vi "sv_Convert Timestamp to Relative Index.vi"(7 "waveform dt":dbl, 10 "timestamp":timestamp, 11 "waveform timestamp":timestamp) -> (2 "Y index":i32)   [LabVIEW 2017]
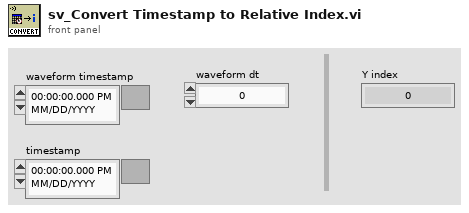
[diagram p1: front panel]
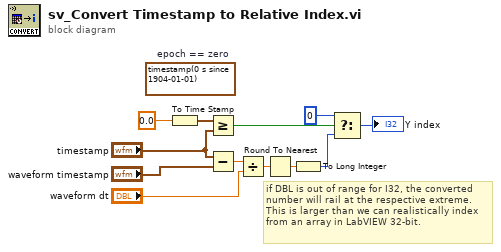
[diagram p0: block diagram]
diagram:
  (unwired) timestamp(0 s since 1904-01-01)  # epoch == zero
  # "if DBL is out of range for I32, the converted number will rail at the respective extreme. This is larger than we can realistically index from an array in LabVIEW 32-bit."
  n1 = To Time Stamp(1:0.0 ("number")) -> (0:w1:timestamp)
  n2 = Greater Or Equal?(x=w1, y="timestamp") -> (x >= y?=w11:bool)
  n3 = Subtract(x="timestamp", y="waveform timestamp") -> (x-y=w7:dbl)
  n4 = Divide(x=w7, y="waveform dt") -> (x/y=w10:dbl)
  n5 = Round To Nearest(number=w10) -> (nearest integer value=w9:dbl)
  n6 = To Long Integer(number=w9) -> (32bit integer=w6:i32)
  n7 = Select(t=0, s=w11, f=w6) -> (s? t:f=→"Y index":i32)
